vi "Normalisation.vi"(1 "Input Time Serie [V]":dbl[](array[numeric])) -> (0 "Normalised Time Serie [\\]":dbl[](array[numeric]))   [LabVIEW 2023]
doc: "Simple VI for normalising data in the range (0,1). The final value is calculated as:\nVout(i) = /V(i) - Vmin) / (Vmax - Vmin); where Vmin e Vmax sono rispettivamente il minimo e il massimo valore dell'arrey\nInputs:\n- Time serie\nOutputs:\n- Normalised Time series"
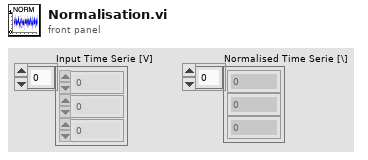
[diagram p1: front panel]
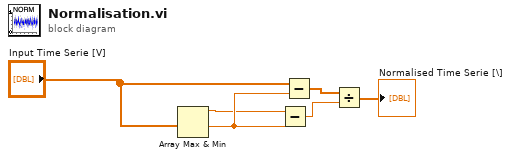
[diagram p0: block diagram]
diagram:
  n1 = Array Max & Min(array="Input Time Serie [V]") -> (max value=w2:dbl, min value=w4:dbl)  [unwired: 2 out]
  n2 = Subtract(x=w2, y=w4) -> (x-y=w6:dbl)
  n3 = Subtract(x="Input Time Serie [V]", y=w4) -> (x-y=w5:dbl[])
  n4 = Divide(x=w5, y=w6) -> (x/y=→"Normalised Time Serie [\\]":dbl[])
